vi "PRIME Detector Wait for Command to Complete.vi"(8 "error in (no error)":errorcluster, 9 "Exp Time":dbl=60.0, 10 "timeout (120s)":dbl=120.0, 11 "connection ID":refnum<k5>) -> (0 "error out":errorcluster, 2 "Status":T1, 3 "connection ID out":refnum<k5>)   [LabVIEW 2021, in "PRIME Detector.lvclass"]
uses:
  PRIME Detector.lvclass
  PRIME Detector cluster Status.ctl
panel:
  out "Time Remaining":dbl(knob) scale=-1.0..10.0
  out "Command":string
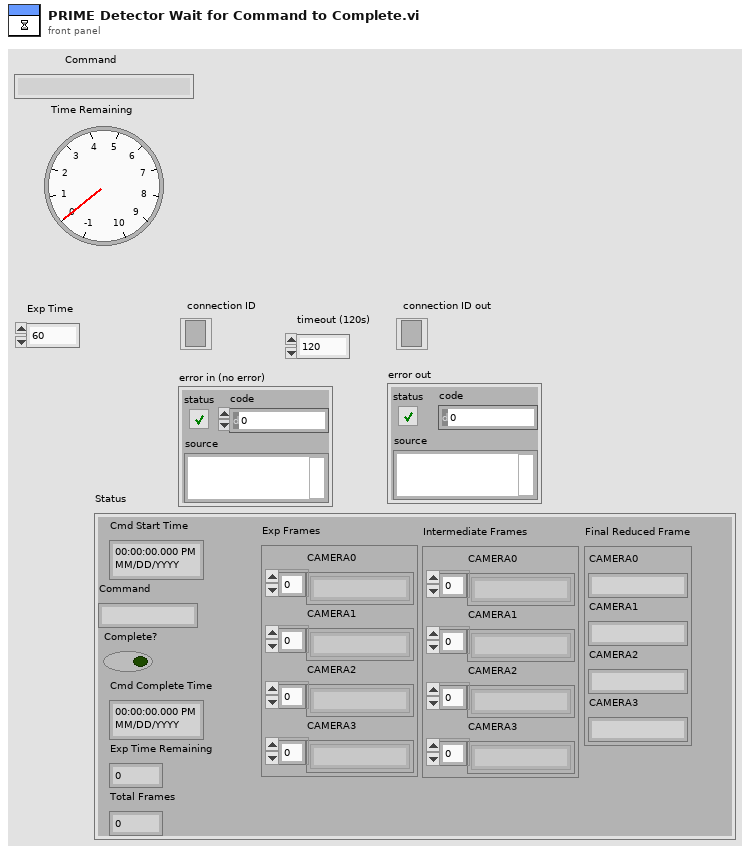
[diagram p1: front panel]
types:
  T1 = typedef "PRIME Detector cluster Status.ctl" = cluster{"Cmd Start Time":timestamp, "Command":string, "Complete?":bool, "Cmd Complete Time":timestamp, "Exp Time Remaining":dbl, "Total Frames":i32, "Exp Frames":cluster{"CAMERA0":string[], "CAMERA1":string[], "CAMERA2":string[], "CAMERA3":string[]}, "Intermediate Frames":cluster{"CAMERA0":string[], "CAMERA1":string[], "CAMERA2":string[], "CAMERA3":string[]}, "Final Reduced Frame":cluster{"CAMERA0":string, "CAMERA1":string, "CAMERA2":string, "CAMERA3":string}}
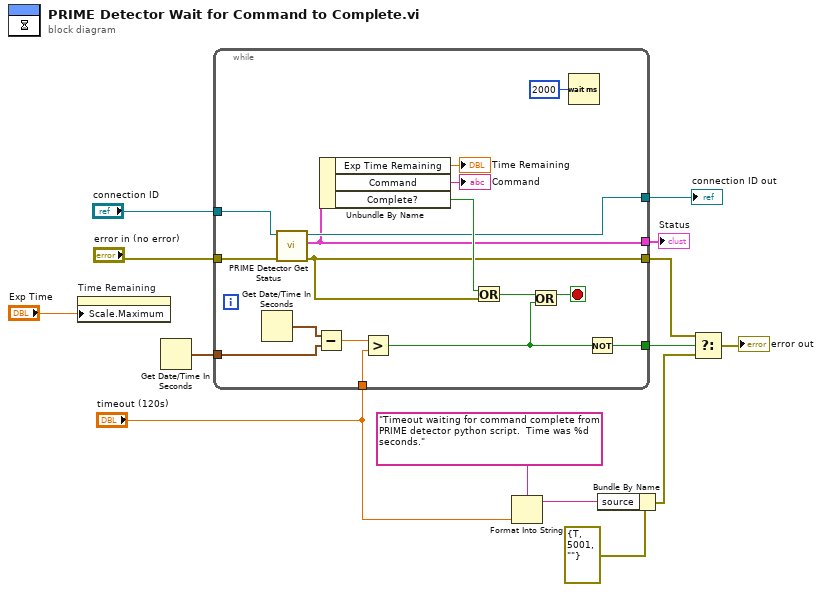
[diagram p0: block diagram]
diagram:
  n1 = property on="Time Remaining" class="Knob (strict)"("Scale.Maximum"="Exp Time") -> ()  [unwired: 2 in, 2 out]
  n2 = Get Date/Time In Seconds() -> (seconds since 1Jan1904=w12:timestamp)
  n3 = while {
    tunnel: "error in (no error)" -> [w31]
    tunnel: "connection ID" -> [w30]
    tunnel: [w27] -> w7
    tunnel: w12 -> [w24]
    tunnel: "timeout (120s)" -> [w22]
    tunnel: [w19] -> w10
    tunnel: [w18] -> w9
    tunnel: [w15] -> w8
    stop <- w17 stop-if-true
    n4 = Get Date/Time In Seconds() -> (seconds since 1Jan1904=w25:timestamp)
    n5 = call "PRIME Detector Get Status.vi"("error in (no error)"=w31, "connection ID"=w30) -> ("error out"=w27:errorcluster, "Status"=w18:T1, "connection ID out"=w19:refnum<k5>)  [unwired: 6 in, 1 out]
    n6 = Subtract(x=w25, y=w24) -> (x-y=w23:dbl)
    n7 = Unbundle By Name(w18) -> ("Exp Time Remaining"=→"Time Remaining":dbl, "Command"=→"Command":string, "Complete?"=w29:bool)
    n8 = Greater?(x=w23, y=w22) -> (0:w16:bool)
    n9 = Or(x=w29, y=w27) -> (x .or. y?=w28:bool)
    n10 = Or(x=w28, y=w16) -> (x .or. y?=w17:bool)
    n11 = Wait (ms)(milliseconds to wait=u32 2000 ("millisecond multiple")) -> ()  [unwired: 1 out]
    n12 = Not(x=w16) -> (.not. x?=w15:bool)
  }
  "connection ID out" <- w10
  "Status" <- w9
  n13 = Format Into String(format string="Timeout waiting for command complete from PRIME detector python script.  Time was %d seconds." ("source"), "timeout (120s)") -> (resulting string=w2:string)  [unwired: 2 in, 1 out]
  n14 = Bundle By Name(cluster=errorcluster {"status"=TRUE, "code"=5001, "source"=""} ("f"), "source"=w2) -> (w1:errorcluster)
  n15 = Select(t=w7, s=w8, f=w1) -> (s? t:f=→"error out":errorcluster)
